vi "Update Config Tree.vi"(8 "error in (no error)":errorcluster, 10 "devices":refnum<vi>, 11 "session in":refnum<k21>) -> (0 "error out":errorcluster, 2 "devices out":refnum<vi>, 3 "session out":refnum<k21>)   [LabVIEW 2017]
uses:
  <resource>/objmgr/slsc.rc
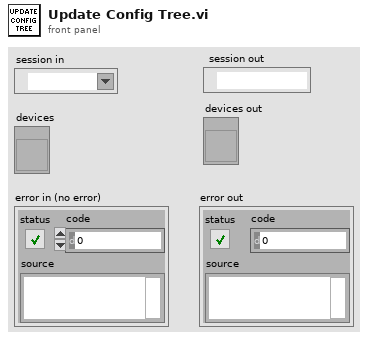
[diagram p1: front panel]
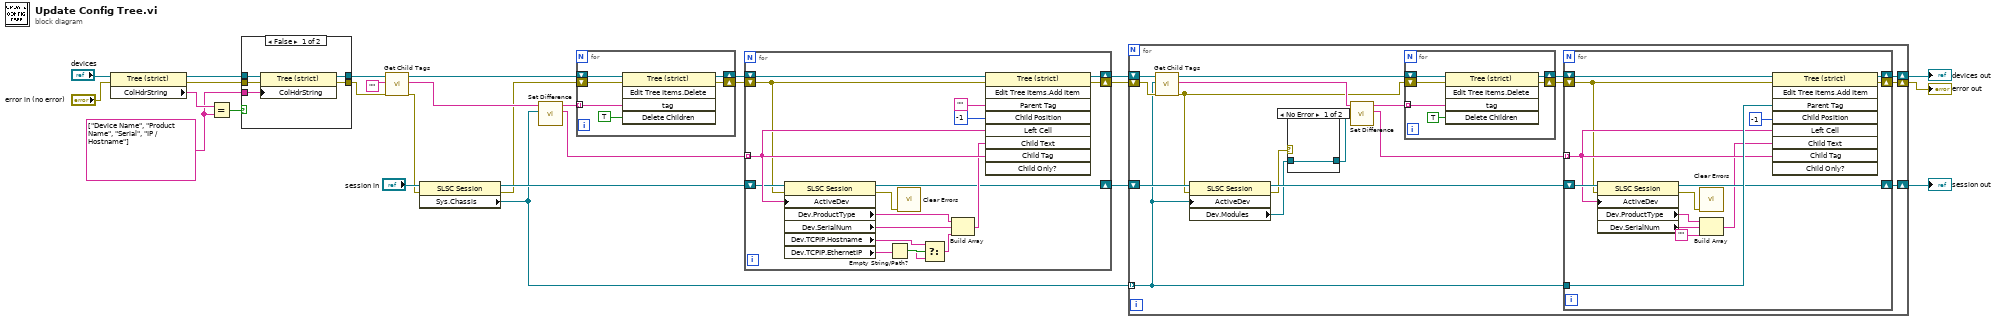
[diagram p0: block diagram]
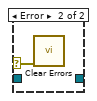
[diagram p2: hidden frame]
diagram:
  w1 = string[] ["Device Name", "Product Name", "Serial", "IP / Hostname"]
  n1 = property class="Tree (strict)"(reference="devices", error in="error in (no error)") -> (reference out=w24:refnum<vi>, error out=w23:errorcluster, "ColHdrString"=w26:string[])
  n2 = Equal?(x=w26, y=w1) -> (x = y?=w25:bool)
  n3 = case shown="False" w25 {
    tunnel: w24 -> [w32 w34]
    tunnel: w23 -> [w31 w33]
    tunnel: w1 -> [w30 _]
    tunnel: [w29 w33] -> w21
    tunnel: [w28 w34] -> w22
    frame False {
      n4 = property class="Tree (strict)"(reference=w32, error in=w31, "ColHdrString"=w30) -> (reference out=w28:refnum<vi>, error out=w29:errorcluster)
    }
    frame True {
    }
  }
  n5 = call "Get Child Tags.vi"("error in (no error)"=w21, "parent tag"="", "tree in"=w22) -> ("error out"=w4:errorcluster, "child tags"=w18:string[], "tree out"=w17:refnum<vi>)  [unwired: 6 in]
  n6 = property class="SLSC Session"(reference="session in", error in=w4) -> (reference out=w5:refnum<k21>, error out=w3:errorcluster, "Sys.Chassis"=w2:refnum<k21>[])
  n7 = call "Set Difference.vi"("b"=w2, "a"=w18) -> ("b - a"=w7:string[], "a - b"=w8:string[])  [unwired: 8 in]
  n8 = for {
    tunnel: w8 -> [w40] mode=indexing
    shift-right: [w37] -> w16
    shift-left: w17 -> [w38]
    shift-right: [w35] -> w15
    shift-left: w3 -> [w36]
    n9 = invoke class="Tree (strict)" method="Edit Tree Items.Delete"(reference=w38, error in=w36, "tag"=w40, "Delete Children"=TRUE ("Delete Children?")) -> (reference out=w37:refnum<vi>, error out=w35:errorcluster)  [unwired: 1 in, 3 out]
  }
  n10 = for {
    tunnel: w7 -> [w52] mode=indexing
    shift-right: [w48] -> w14
    shift-left: w5 -> [w49]
    shift-right: [w54] -> w12
    shift-left: w16 -> [w55]
    shift-right: [w53] -> w13
    shift-left: w15 -> [w47]
    n11 = property class="SLSC Session"(reference=w49, error in=w47, "ActiveDev"=w52) -> (reference out=w48:refnum<k21>, error out=w41:errorcluster, "Dev.ProductType"=w51:string, "Dev.SerialNum"=w43:string, "Dev.TCPIP.Hostname"=w46:string, "Dev.TCPIP.EthernetIP"=w44:string)
    n12 = Empty String/Path?(string/path=w44) -> (empty?=w45:bool)
    n13 = call <vilib>:"Clear Errors.vi"("error in (no error)"=w41) -> ()  [unwired: 5 in, 2 out]
    n14 = Select(t=w46, s=w45, f=w44) -> (s? t:f=w42:string)
    n15 = Build Array(w51, w43, w42) -> (w50:string[])
    n16 = invoke on="Invoke Node" class="Tree (strict)" method="Edit Tree Items.Add Item"(reference=w55, error in=w47, "Parent Tag"="", "Child Position"=-1, "Left Cell"=w52, "Child Text"=w50, "Child Tag"=w52) -> (reference out=w54:refnum<vi>, error out=w53:errorcluster)  [unwired: 2 in, 7 out]
  }
  n17 = for {
    tunnel: w2 -> [w63] mode=indexing
    shift-right: [w67] -> w11
    shift-left: w14 -> [w64]
    shift-right: [w70] -> w9
    shift-left: w13 -> [w71]
    shift-right: [w68] -> w10
    shift-left: w12 -> [w69]
    n18 = call "Get Child Tags.vi"("error in (no error)"=w71, "parent tag"=w63, "tree in"=w69) -> ("error out"=w58:errorcluster, "child tags"=w75:string[], "tree out"=w74:refnum<vi>)  [unwired: 6 in]
    n19 = property class="SLSC Session"(reference=w64, error in=w58, "ActiveDev"=w63) -> (reference out=w62:refnum<k21>, error out=w61:errorcluster, "Dev.Modules"=w60:refnum<k21>[])
    n20 = case shown="No Error" w61 {
      selector: w61 -> [_ w77]
      tunnel: [w76 _] -> w59
      tunnel: w60 -> [w76 _]
      frame No Error {
      }
      frame Error {
        n21 = call <vilib>:"Clear Errors.vi"("error in (no error)"=w77) -> ()  [unwired: 5 in, 2 out]
      }
    }
    n22 = call "Set Difference.vi"("b"=w59, "a"=w75) -> ("b - a"=w65:string[], "a - b"=w66:string[])  [unwired: 8 in]
    n23 = for {
      tunnel: w66 -> [w97] mode=indexing
      shift-right: [w94] -> w73
      shift-left: w74 -> [w95]
      shift-right: [w92] -> w72
      shift-left: w58 -> [w93]
      n24 = invoke class="Tree (strict)" method="Edit Tree Items.Delete"(reference=w95, error in=w93, "tag"=w97, "Delete Children"=TRUE ("Delete Children?")) -> (reference out=w94:refnum<vi>, error out=w92:errorcluster)  [unwired: 1 in, 3 out]
    }
    n25 = for {
      shift-right: [w86] -> w67
      shift-left: w62 -> [w87]
      shift-right: [w90] -> w68
      shift-left: w73 -> [w78]
      shift-right: [w89] -> w70
      shift-left: w72 -> [w82]
      tunnel: w65 -> [w84] mode=indexing
      tunnel: w63 -> [w88]
      n26 = property class="SLSC Session"(reference=w87, error in=w82, "ActiveDev"=w84) -> (reference out=w86:refnum<k21>, error out=w79:errorcluster, "Dev.ProductType"=w85:string, "Dev.SerialNum"=w81:string)
      n27 = call <vilib>:"Clear Errors.vi"("error in (no error)"=w79) -> ()  [unwired: 5 in, 2 out]
      n28 = Build Array(w85, w81, "") -> (w83:string[])
      n29 = invoke on="Invoke Node" class="Tree (strict)" method="Edit Tree Items.Add Item"(reference=w78, error in=w82, "Parent Tag"=w88, "Child Position"=-1, "Left Cell"=w84, "Child Text"=w83, "Child Tag"=w84) -> (reference out=w90:refnum<vi>, error out=w89:errorcluster)  [unwired: 2 in, 7 out]
    }
  }
  "error out" <- w9
  "devices out" <- w10
  "session out" <- w11
